vi "Trap Density.vi"(9 "Temp (T) [K]":dbl, 10 "S.T.S. (S)":dbl, 11 "Capacitance (C)":dbl) -> (3 "Trap Density (N)":dbl)   [LabVIEW 2011]
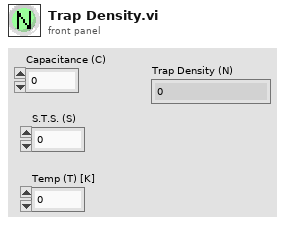
[diagram p1: front panel]
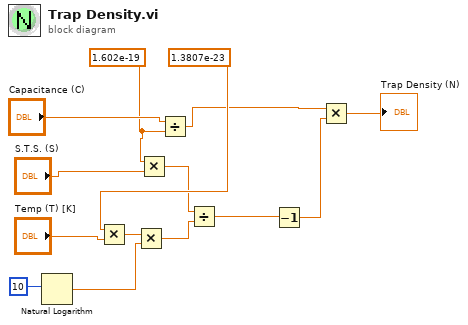
[diagram p0: block diagram]
diagram:
  w12 = 1.602e-19
  n1 = Natural Logarithm(1:10) -> (0:w6:dbl)
  n2 = Multiply(x=1.3807e-23, y="Temp (T) [K]") -> (x*y=w7:dbl)
  n3 = Multiply(x=w7, y=w6) -> (x*y=w4:dbl)
  n4 = Multiply(x=w12, y="S.T.S. (S)") -> (x*y=w5:dbl)
  n5 = Divide(x="Capacitance (C)", y=w12) -> (x/y=w2:dbl)
  n6 = Divide(x=w5, y=w4) -> (x/y=w3:dbl)
  n7 = Decrement(x=w3) -> (x-1=w1:dbl)
  n8 = Multiply(x=w2, y=w1) -> (x*y=→"Trap Density (N)":dbl)
